vi "blinking_button.vi"() -> ()   [LabVIEW 2021]
panel:
  in  "stop":bool
  in  "Knob":dbl(knob) scale=0.0..10.0
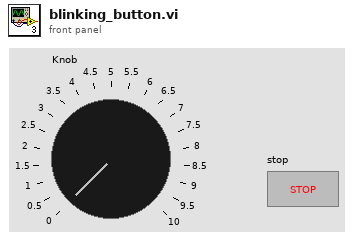
[diagram p1: front panel]
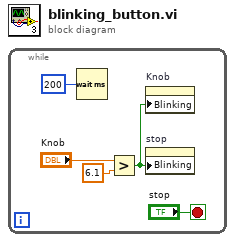
[diagram p0: block diagram]
diagram:
  n1 = while {
    stop <- "stop" stop-if-true
    n2 = Wait (ms)(milliseconds to wait=u32 200) -> ()  [unwired: 1 out]
    n3 = Greater?(x="Knob", y=6.1) -> (0:w1:bool)
    n4 = property on="Knob" class="Knob (strict)"("Blinking"=w1) -> ()  [unwired: 2 in, 2 out]
    n5 = property on="stop" class="Bool"("Blinking"=w1) -> ()  [unwired: 2 in, 2 out]
  }
